vi "FOURIER TRANSLATION.vi"() -> ()   [LabVIEW 2018]
uses:
  <vilib>/express/express analysis/Spectral/Block/exnSpectralBlock spectral measurements RMS poly.vi
  <vilib>/express/express analysis/Spectral/Block/exnSpectralBlock spectral measurements RMS DDT.vi
  <vilib>/express/express analysis/Spectral/XNode/ExpressSpectralMeasurementsBlockNode.xnode
panel:
  out "Waveform Graph":dynamicdata(graph)
  in  "stop":bool
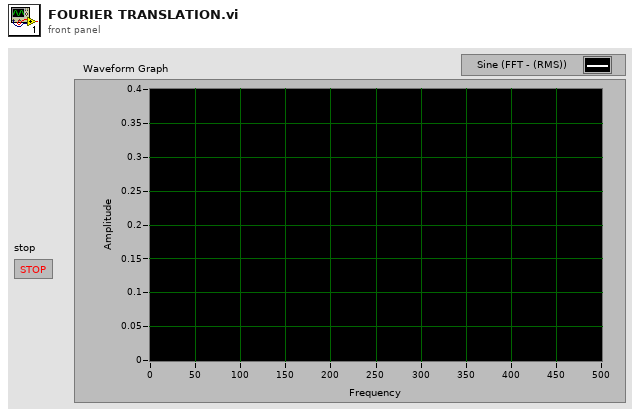
[diagram p1: front panel]
types:
  T1 = cluster{"averaging mode":u16, "weighting mode":u16, "number of averages":u32}
  T2 = cluster{"dB On (F)":bool, "unwrap phase (F)":bool, "convert to degree (F)":bool}
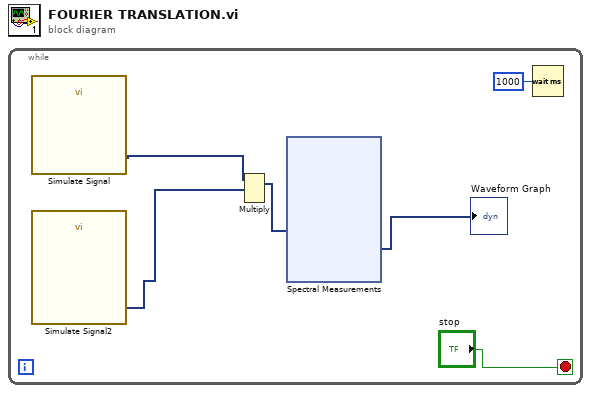
[diagram p0: block diagram]
diagram:
  n1 = while {
    stop <- "stop" stop-if-true
    n2 = call "Simulate Signal"() -> ("Sine"=w1:dynamicdata)  [unwired: 14 in, 1 out]
    n3 = call "Simulate Signal2"() -> ("Sine"=w2:dynamicdata)  [unwired: 14 in, 1 out]
    n4 = Multiply(1:w2, 2:w1) -> (0:w3:dynamicdata)  [unwired: 1 in, 1 out]
    n5 = xnode "Spectral Measurements"("Signals"=w3) -> ("FFT - (RMS)"=→"Waveform Graph":dynamicdata)  [unwired: 1 in, 2 out]
    n6 = Wait (ms)(milliseconds to wait=u32 1000) -> ()  [unwired: 1 out]
  }
